vi "InitSeeSaw.vi"(8 "error in (no error)":errorcluster, 11 "AdaFruit-Seesaw in":refnum<class "AdaFruit-Seesaw.lvclass">) -> (0 "error out":errorcluster, 1 "Date":u16, 2 "Version":u16, 3 "AdaFruit-Seesaw out":refnum<class "AdaFruit-Seesaw.lvclass">, 5 "HW_ID":string)   [LabVIEW 2020, in "CTI-Peripheral.lvlib" / "AdaFruit-Seesaw.lvclass"]
uses:
  AdaFruit-Seesaw.lvclass
  AdaFruit-Seesaw.lvclass/AdaFruit-Seesaw.ctl
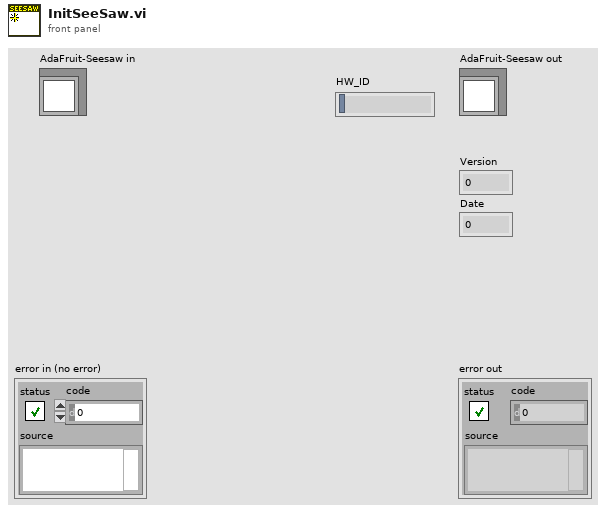
[diagram p1: front panel]
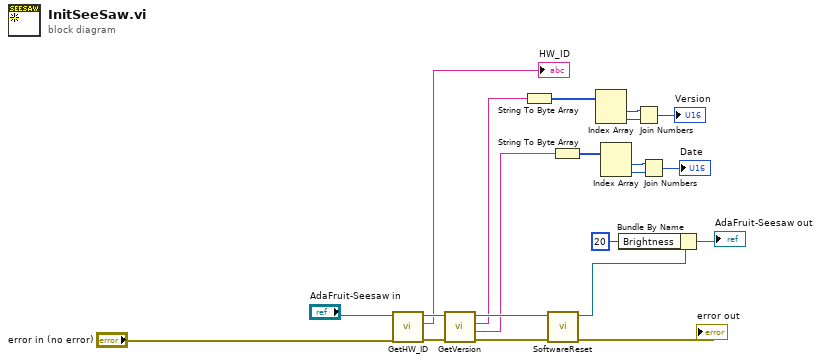
[diagram p0: block diagram]
diagram:
  n1 = call "GetHW_ID.vi"("error in (no error)"="error in (no error)", "AdaFruit-Seesaw in"="AdaFruit-Seesaw in") -> ("error out"=w17:errorcluster, "HW_ID"=→"HW_ID":string, "AdaFruit-Seesaw out"=w20:refnum<class "AdaFruit-Seesaw.lvclass">)  [unwired: 7 in]
  n2 = call "GetVersion.vi"("error in (no error)"=w17, "AdaFruit-Seesaw in"=w20) -> ("error out"=w18:errorcluster, "DateCode"=w6:string, "Version"=w14:string, "AdaFruit-Seesaw out"=w19:refnum<class "AdaFruit-Seesaw.lvclass">)  [unwired: 6 in]
  n3 = String To Byte Array(string=w14) -> (unsigned byte array=w13:u8[])
  n4 = call "SoftwareReset.vi"("error in (no error)"=w18, "AdaFruit-Seesaw in"=w19) -> ("error out"=→"error out":errorcluster, "AdaFruit-Seesaw out"=w3:refnum<class "AdaFruit-Seesaw.lvclass">)  [unwired: 8 in]
  n5 = String To Byte Array(string=w6) -> (unsigned byte array=w5:u8[])
  n6 = Index Array(array=w13) -> (element #1=w11:u8, element #2=w12:u8)  [unwired: 2 in]
  n7 = Index Array(array=w5) -> (element #1=w8:u8, element #2=w7:u8)  [unwired: 2 in]
  n8 = Bundle By Name(cluster=w3, "Brightness"=u8 20) -> (→"AdaFruit-Seesaw out":refnum<class "AdaFruit-Seesaw.lvclass">)
  n9 = Join Numbers(hi=w11, lo=w12) -> ((hi.lo)=→"Version":u16)
  n10 = Join Numbers(hi=w8, lo=w7) -> ((hi.lo)=→"Date":u16)
